vi "Get Owning Library QD.vi"(8 "error in (no error)":errorcluster, 11 "VI in":refnum<vi>) -> (0 "error out":errorcluster, 1 "Not In Library":bool, 2 "Owning Library":refnum<vi>, 3 "VI out":refnum<vi>)   [LabVIEW 2017]
doc: "Returns the owning library of the selected VI."
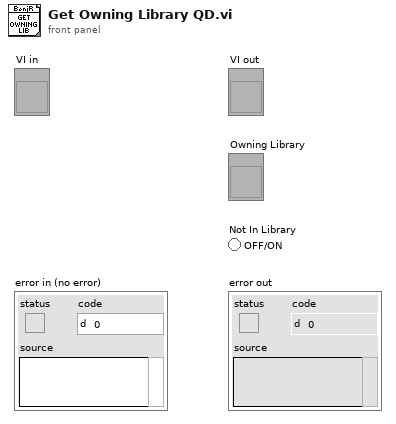
[diagram p1: front panel]
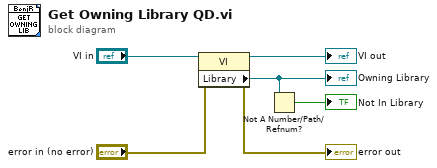
[diagram p0: block diagram]
diagram:
  n1 = property class="VI"(reference="VI in", error in="error in (no error)") -> (reference out=→"VI out":refnum<vi>, error out=→"error out":errorcluster, "Library"=w2:refnum<vi>)
  "Owning Library" <- w2
  n2 = Not A Number/Path/Refnum?(number/path/refnum=w2) -> (NaN/Path/Refnum?=→"Not In Library":bool)
